vi "Destroy.vi"(0 "reference in":refnum<class "SSR.lvclass">, 5 "error in (no error)":errorcluster) -> (14 "reference out":refnum<class "SSR.lvclass">, 19 "error out":errorcluster)   [LabVIEW 2017, in "SSR.lvclass"]
uses:
  SSR.lvclass
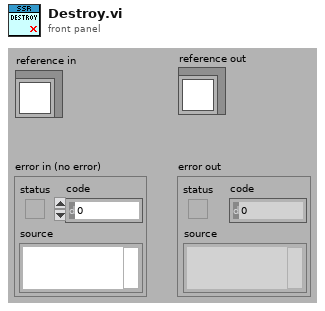
[diagram p1: front panel]
types:
  T1 = typedef "SSR.lvclass/ObjectAttributes.ctl" = cluster{"SSR Task":refnum<k21>, "SSR On/Off Status":bool, "Number of SSR Modules":u32, "Number of Total SSR Channels":u32, "SSR Module Names (NI-Max Name)":string[], "Number of Channels Per SSR Module":i32[], "SSR Status":bool[], "SSR Status to Set":bool[], "SSR VI Reference":refnum<vi>}
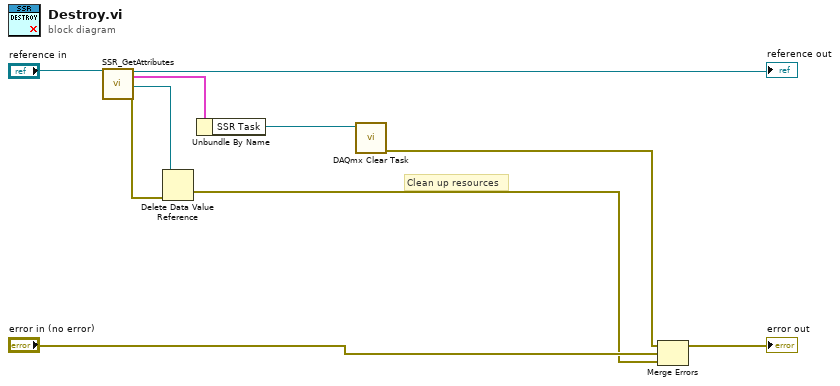
[diagram p0: block diagram]
diagram:
  # "Clean up resources"
  n1 = call "SSR_GetAttributes.vi"("reference in"="reference in") -> ("reference out"=→"reference out":refnum<class "SSR.lvclass">, "Data"=w5:T1, "DataRef"=w6:refnum<data-value>, "error out"=w7:errorcluster)  [unwired: 15 in]
  n2 = Delete Data Value Reference(data value reference=w6, error in=w7) -> (error out=w3:errorcluster)  [unwired: 1 out]
  n3 = Unbundle By Name(w5) -> ("SSR Task"=w2:refnum<k21>)
  n4 = call <vilib>:"DAQmx Clear Task.vi"("task in"=w2) -> ("error out"=w1:errorcluster)  [unwired: 14 in]
  n5 = Merge Errors(w1, "error in (no error)", w3) -> (→"error out":errorcluster)
